vi "SoundToFileEntry.vi"() -> ()   [LabVIEW 2015]
uses:
  <vilib>/sound2/lvsound2.llb/Sound Data Format.ctl
  <vilib>/sound2/lvsound2.llb/Sampling Mode.ctl
  <vilib>/sound2/lvsound2.llb/Sound File Write Open.vi
  <vilib>/sound2/lvsound2.llb/Sound Input Read (DBL).vi
  <vilib>/sound2/lvsound2.llb/Sound File Write (DBL).vi
panel:
  in  "stop":bool
  in  "sound format":T1={"sample rate (S/s)"=22050.0, "number of channels"=2, "bits per sample"=16}
  in  "device ID":u32
  in  "number of samples/ch":i32=100000
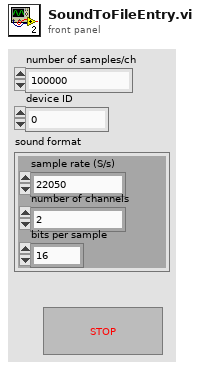
[diagram p1: front panel]
types:
  T1 = typedef "Sound Data Format.ctl" = cluster{"sample rate (S/s)":dbl, "number of channels":i32, "bits per sample":i32}
  T2 = typedef "Sampling Mode.ctl" = i32
  T3 = typedef "Sound File Refnum.ctl" = refnum<file>
  T4 = typedef "Sound Input Task ID.ctl" = u32
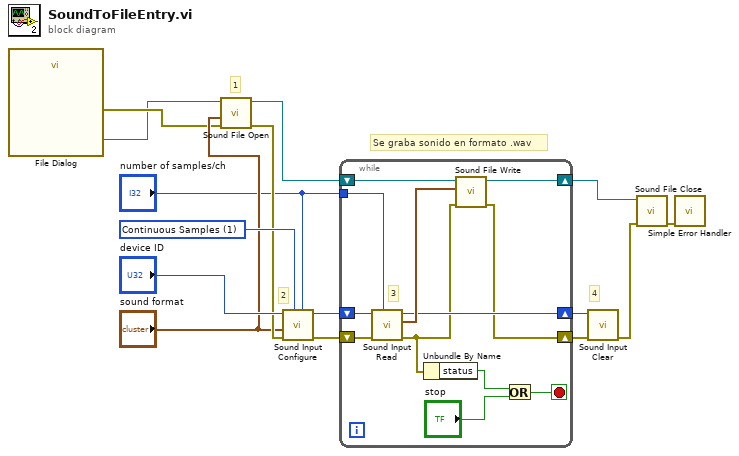
[diagram p0: block diagram]
diagram:
  w15 = T2 1 items=["Finite Samples", "Continuous Samples"] ("sample mode")
  # "Se graba sonido en formato .wav"
  # "4"
  # "2"
  # "1"
  n1 = call "File Dialog"() -> ("selected path"=w1:path, "error out"=w2:errorcluster)  [unwired: 12 in, 2 out]
  n2 = call-poly <vilib>:"Sound File Open.vi"("error in (no error)"=w2, "sound format"="sound format", "path"=w1) -> ("error out"=w13:errorcluster, "sound file refnum"=w8:T3)  [unwired: 7 in]
  n3 = call <vilib>:"Sound Input Configure.vi"("number of samples/ch"="number of samples/ch", "sample mode"=w15, "error in (no error)"=w13, "sound format"="sound format", "device ID"="device ID") -> ("error out"=w10:errorcluster, "task ID"=w11:T4)  [unwired: 5 in]
  n4 = while {
    tunnel: "number of samples/ch" -> [w25]
    shift-right: [w23] -> w5
    shift-left: w8 -> [w24]
    shift-right: [w21] -> w6
    shift-left: w11 -> [w26]
    shift-right: [w20] -> w7
    shift-left: w10 -> [w27]
    stop <- w16 stop-if-true
    # "3"
    n5 = call-poly <vilib>:"Sound Input Read.vi"("number of samples/ch"=w25, "error in (no error)"=w27, "task ID"=w26) -> ("error out"=w19:errorcluster, "data"=w22:waveform(dbl)[], "task ID out"=w21:T4)  [unwired: 6 in]
    n6 = Unbundle By Name(w19) -> ("status"=w18:bool)
    n7 = call-poly <vilib>:"Sound File Write.vi"("error in (no error)"=w19, "data"=w22, "sound file refnum"=w24) -> ("error out"=w20:errorcluster, "sound file refnum out"=w23:T3)  [unwired: 7 in]
    n8 = Or(x=w18, y="stop") -> (x .or. y?=w16:bool)
  }
  n9 = call <vilib>:"Sound Input Clear.vi"("error in (no error)"=w7, "task ID"=w6) -> ("error out"=w4:errorcluster)  [unwired: 9 in]
  n10 = call <vilib>:"Sound File Close.vi"("error in (no error)"=w4, "sound file refnum"=w5) -> ("error out"=w3:errorcluster)  [unwired: 9 in]
  n11 = call <vilib>:"Simple Error Handler.vi"("error in (no error)"=w3) -> ()  [unwired: 4 in, 5 out]
